vi "Read Core.vi"(8 "error in (no error)":errorcluster, 9 "Timeout (1s)":dbl[unit]=1.0, 11 "DIMConnection in":refnum<class "DIMConnection.lvclass">) -> (0 "error out":errorcluster, 1 "timed out":bool, 2 "PV":refnum<class "PV.lvclass">, 3 "DIMConnection out":refnum<class "DIMConnection.lvclass">)   [LabVIEW 2014, in "CS++DIM.lvlib" / "DIMConnection.lvclass"]
doc: "Read a process varibale."
uses:
  DIMConnection.lvclass
  DimLVEvent/LVDimInterface/LVDimInterface.lvlib
  CSPP_Core/Classes/CS++ProcessVariables/PVConnection/PVConnection.lvclass
  CSPP_Core/Classes/CS++ProcessVariables/ProcessVariable/PV.lvclass
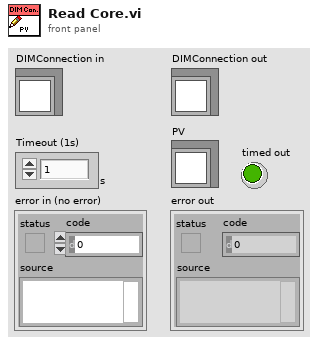
[diagram p1: front panel]
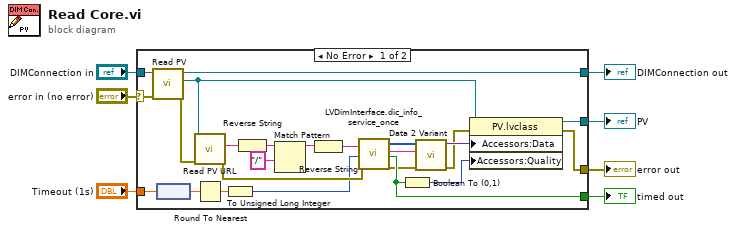
[diagram p0: block diagram]
diagram:
  n1 = case shown="No Error" "error in (no error)" {
    selector: "error in (no error)" -> [w18 w32]
    tunnel: "DIMConnection in" -> [w31 w33]
    tunnel: [w30 w33] -> w6
    tunnel: [w21 _] -> w5
    tunnel: [w20 w32] -> w4
    tunnel: [w17 _] -> w2
    tunnel: "Timeout (1s)" -> [w15 _]
    frame No Error {
      n2 = call "Read PV.vi"("error in (no error)"=w18, "PVConnection in"=w31) -> ("error out"=w29:errorcluster, "PV"=w22:refnum<class "PV.lvclass">, "PVConnection out"=w30:refnum<class "DIMConnection.lvclass">)  [unwired: 7 in]
      n3 = node(w15) -> (w16:dbl)
      n4 = call "Read PV URL.vi"("error in (no error)"=w29, "PV in"=w22) -> ("error out"=w23:errorcluster, "PV URL"=w28:string)  [unwired: 7 in, 1 out]
      n5 = Round To Nearest(number=w16) -> (nearest integer value=w14:dbl)
      n6 = To Unsigned Long Integer(number=w14) -> (unsigned 32bit integer=w13:u32)
      n7 = Reverse String(1:w28) -> (0:w27:string)
      n8 = Match Pattern(string=w27, regular expression="/") -> (before substring=w25:string)  [unwired: 1 in, 3 out]
      n9 = Reverse String(1:w25) -> (0:w24:string)
      n10 = call "LVDimInterface.dic_info_service_once.vi"("serviceName"=w24, "timeout [ms]"=w13, "error in (no error)"=w23) -> ("data"=w12:i8[], "typeDescriptor"=w11:string, "timed out?"=w17:bool, "error out"=w10:errorcluster)  [unwired: 13 in]
      n11 = Boolean To (0,1)(Boolean=w17) -> (0, 1=w19:i16)
      n12 = call "Data 2 Variant.vi"("Error In"=w10, "Type Descriptor"=w11, "Data"=w12) -> ("Error Out"=w8:errorcluster, "data"=w9:variant)  [unwired: 7 in]
      n13 = property class="PV.lvclass"(reference=w22, error in=w8, "Accessors:Data"=w9, "Accessors:Quality"=w19) -> (reference out=w21:refnum<class "PV.lvclass">, error out=w20:errorcluster)
    }
    frame Error {
    }
  }
  "error out" <- w4
  "DIMConnection out" <- w6
  "PV" <- w5
  "timed out" <- w2
